vi "Init.vi"(4 "Message Cfg":T2={"EnTermChar"=FALSE, "termChar"=10, "suppEnEnRd"=TRUE, "sendEndEn"=FALSE} {"termChar" format="%.0x"}, 6 "timeout":u32=1000, 7 "Name":string="3022A", 8 "error in":errorcluster, 9 "serialCfg":T1={"baud rate (9600)"=9600, "data bits (8)"=7, "stop bits (10: 1 bit)"=10, "parity (0:none)"=enum."Even", "flow control (0:none)"=0, "endModeforReads"=0, "endModeforWrites"=0} {"endModeforWrites" items=["None", "Last Bit", "TermChar", "Break"]; "endModeforReads" items=["None", "Last Bit", "TermChar"]; "flow control (0:none)" items=["None", "XON/XOFF", "RTS/CTS", "XON/XOFF & RTS/CTS", "DTR/DSR", "XON/XOFF & DTR/DSR"]; "stop bits (10: 1 bit)" items=["1.0"=10, "1.5"=15, "2.0"=20]; "data bits (8)" min=5 max=8 step=1}, 10 "Port":refnum<visa-resource-name>, 11 "3022A in":refnum<class "3022A.lvclass">) -> (0 "error out":errorcluster, 3 "3022A out":refnum<class "3022A.lvclass">)   [LabVIEW 2014, in "3022A.lvclass"]
uses:
  3022A.lvclass
  CPC.lvclass
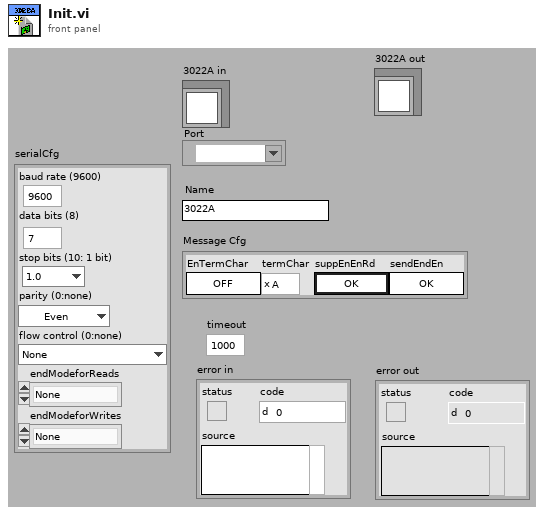
[diagram p1: front panel]
types:
  T1 = cluster{"baud rate (9600)":u32, "data bits (8)":u16, "stop bits (10: 1 bit)":u16, "parity (0:none)":enum16{"None", "Odd", "Even", "Mark", "Space"}, "flow control (0:none)":u16, "endModeforReads":u16, "endModeforWrites":u16}
  T2 = cluster{"EnTermChar":bool, "termChar":u8, "suppEnEnRd":bool, "sendEndEn":bool}
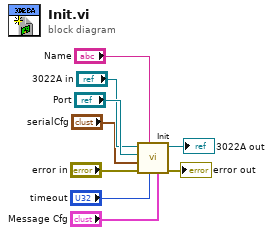
[diagram p0: block diagram]
diagram:
  n1 = call-parent "Init.vi"("Message Cfg"="Message Cfg", "timeout"="timeout", "Name"="Name", "error in"="error in", "serialCfg"="serialCfg", "Port"="Port", "CPC in"="3022A in") -> ("error out"=→"error out":errorcluster, "CPC out"=→"3022A out":refnum<class "3022A.lvclass">)  [unwired: 3 in]
